vi "Get Ambient Temperature.vi"(8 "error in (no error)":errorcluster, 11 "Temperature IR Bricklet in":refnum<class "Temperature IR Bricklet.lvclass">) -> (0 "error out":errorcluster, 2 "Ambient Temperature":i16, 3 "Temperature IR Bricklet out":refnum<class "Temperature IR Bricklet.lvclass">)   [LabVIEW 2011, in "Tinkerforge.lvlib" / "Temperature IR Bricklet.lvclass"]
doc: "This VI returns the ambient temperature value in 1/10 °C."
uses:
  Temperature IR Bricklet.lvclass
  Device/Device.lvclass
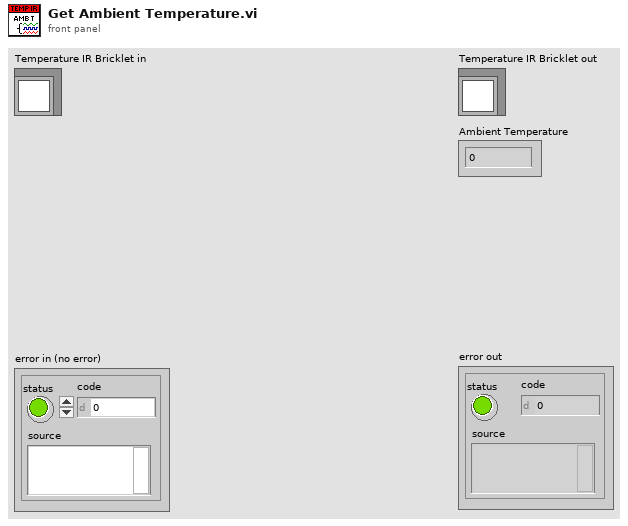
[diagram p1: front panel]
types:
  T1 = typedef "Tinkerforge.lvlib/IP Connection.lvclass/Answer.ctl" = cluster{"Request GUID":string, "Request Type":T2, "Sucessful":bool, "Data":variant, "Error":errorcluster}
  T2 = typedef "Tinkerforge.lvlib/IP Connection.lvclass/Request Type.ctl" = enum8{"Invalid", "Write"}
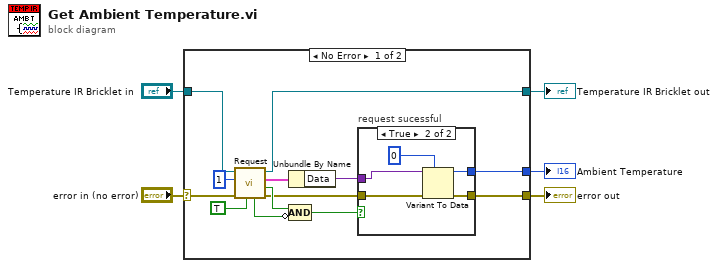
[diagram p0: block diagram]
diagram:
  n1 = case shown="No Error" "error in (no error)" {
    selector: "error in (no error)" -> [w18 w26]
    tunnel: [w7 w26] -> w4
    tunnel: [w16 w25] -> w2
    tunnel: "Temperature IR Bricklet in" -> [w17 w25]
    tunnel: [w6 _] -> w1
    frame No Error {
      n2 = call "Request.vi"("Response"=TRUE, "error in (no error)"=w18, "Function ID"=u8 1, "Device in"=w17) -> ("error out"=w10:errorcluster, "Sucessful"=w12:bool, "Answer"=w9:T1, "Device out"=w16:refnum<class "Temperature IR Bricklet.lvclass">, "timed out"=w13:bool)  [unwired: 3 in]
      n3 = Unbundle By Name(w9) -> ("Data"=w8:variant)
      n4 = Compound Arithmetic op=AND(w12, invert w13) -> (w11:bool)
      n5 = case "request sucessful" shown="True" w11 {
        tunnel: w10 -> [w19 w24]
        tunnel: w8 -> [_ w22]
        tunnel: [_ w21] -> w6
        tunnel: [w19 w20] -> w7
        frame False {
        }
        frame True {
          n6 = Variant To Data(error in=w24, type=i16 0, Variant=w22) -> (data=w21:i16, error out=w20:errorcluster)
        }
      }
    }
    frame Error {
    }
  }
  "error out" <- w4
  "Temperature IR Bricklet out" <- w2
  "Ambient Temperature" <- w1
